vi "Modulator.vi"(8 "error in (no error)":errorcluster, 11 "ISO 15693 DOWN in":refnum<class "ISO 15693 DOWN.lvclass">) -> (0 "error out":errorcluster, 2 "Waveform out":waveform(dbl), 3 "ISO 15693 DOWN out":refnum<class "ISO 15693 DOWN.lvclass">)   [LabVIEW 2019, in "ISO 15693 DOWN.lvclass"]
uses:
  ISO 15693 DOWN.lvclass
  TypeDef/Store.ctl
  ISO 15693 DOWN.lvclass/ISO 15693 DOWN.ctl
  <vilib>/addons/Modulation/Analog/MT Modulate AM (DSB).vi
  <vilib>/addons/Modulation/Analog/MT Upconvert Baseband (Real).vi
  <vilib>/addons/Modulation/niAMT.lvlib
  RFID system.lvclass
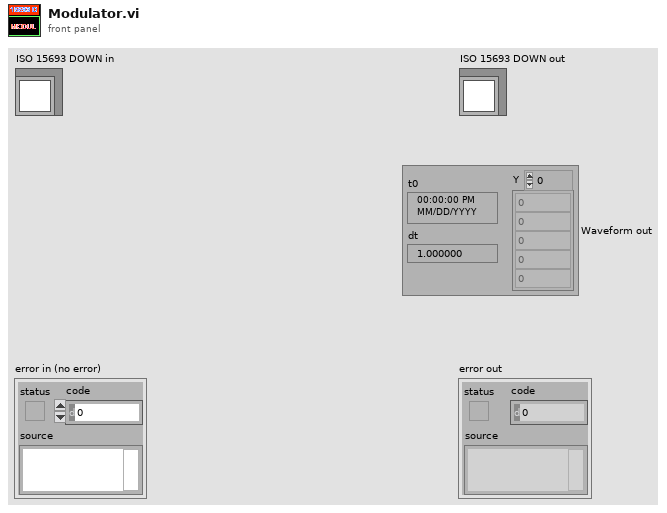
[diagram p1: front panel]
types:
  T1 = typedef "Store.ctl" = enum16{"envelope", "noise", "demSubCar", "CH_frame", "Decode", "demodulate", "in", "out", "sum", "subCarrier", "frame", "command", "encode", "modulate", "encode_UP", "modulate_up", "demod_up", "envelop_up", "sum_up", "out_up", "in_up"}
  T2 = typedef "niAMT.lvlib/Complex Data Waveform.ctl" = cluster{"t0":dbl, "dt":dbl, "Y":cdb[]}
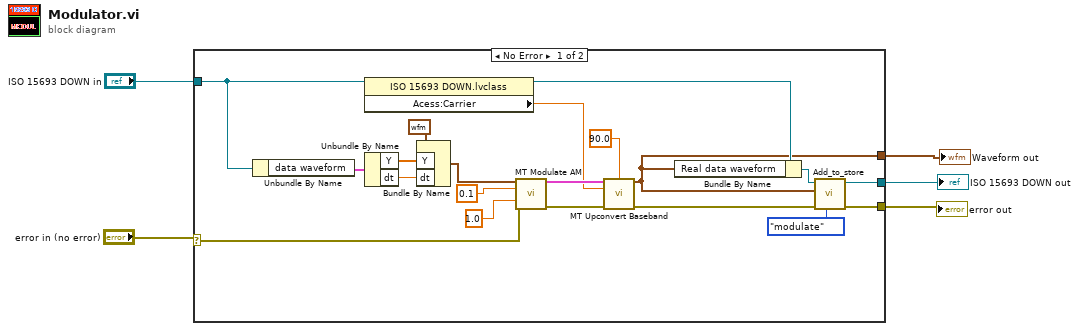
[diagram p0: block diagram]
diagram:
  n1 = case shown="No Error" "error in (no error)" {
    selector: "error in (no error)" -> [w13 w26]
    tunnel: "ISO 15693 DOWN in" -> [w16 w27]
    tunnel: [w9 w27] -> w3
    tunnel: [w8 w26] -> w2
    tunnel: [w6 _] -> w1
    frame No Error {
      n2 = Unbundle By Name(w16) -> ("data waveform"=w15:T2)
      n3 = property class="ISO 15693 DOWN.lvclass"(reference=w16) -> (reference out=w12:refnum<class "ISO 15693 DOWN.lvclass">, "Acess:Carrier"=w14:dbl)  [unwired: 1 in, 1 out]
      n4 = Unbundle By Name(w15) -> ("Y"=w19:cdb[], "dt"=w18:dbl)
      n5 = Bundle By Name(cluster=waveform(cdb) {"t0"=timestamp(0 s since 1904-01-01), "dt"=1.0, "Y"=[]} ("waveform"), "Y"=w19, "dt"=w18) -> (w21:waveform(cdb))
      n6 = call-poly <vilib>:"MT Modulate AM.vi"("message signal"=w21, "modulation index"=0.1, "peak message amplitude"=1.0, "error in (no error)"=w13) -> ("AM modulated waveform"=w20:cluster{"t0":dbl, "dt":dbl, "Y":cdb[]}, "error out"=w23:errorcluster)  [unwired: 10 in]
      n7 = call-poly <vilib>:"MT Upconvert Baseband.vi"("baseband waveform (complex)"=w20, "initial phase (deg)"=90.0, "carrier frequency (Hz)"=w14, "error in (no error)"=w23) -> ("passband waveform"=w6:waveform(dbl), "error out"=w10:errorcluster)  [unwired: 10 in]
      n8 = Bundle By Name(cluster=w12, "Real data waveform"=w6) -> (w11:refnum<class "ISO 15693 DOWN.lvclass">)
      n9 = call "Add_to_store.vi"("Store"=Store."modulate", "error in (no error)"=w10, "Waveform"=w6, "RFID system in"=w11) -> ("error out"=w8:errorcluster, "RFID system out"=w9:refnum<class "ISO 15693 DOWN.lvclass">)  [unwired: 6 in]
    }
    frame Error {
    }
  }
  "error out" <- w2
  "ISO 15693 DOWN out" <- w3
  "Waveform out" <- w1
